vi "Config.vi"(8 "error in":errorcluster, 11 "Instrument Handle In":i32) -> (0 "error out":errorcluster, 2 "Configuration out":i32[](array[numeric]), 3 "Instrument Handle Out":i32)   [LabVIEW 8.6, in "ZTScopeM.lvlib"]
doc: "Query the instrument configuration state."
uses:
  ZTScopeM.lvlib
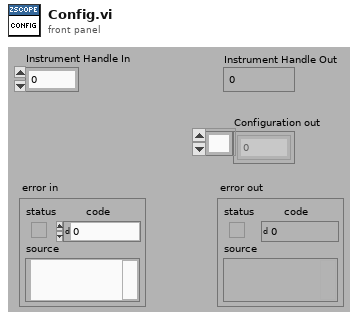
[diagram p1: front panel]
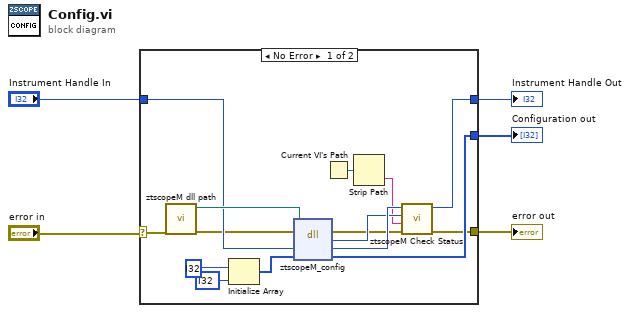
[diagram p0: block diagram]
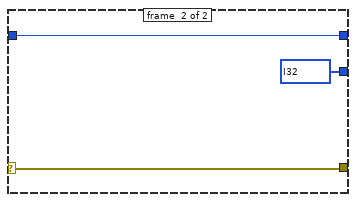
[diagram p2: hidden frame]
diagram:
  n1 = case shown="No Error" "error in" {
    selector: "error in" -> [w10 w23]
    tunnel: [w15 w23] -> w4
    tunnel: [w14 w21] -> w3
    tunnel: [w19 i32[] ? ("Configuration")] -> w2
    tunnel: "Instrument Handle In" -> [w8 w21]
    frame #0 {
      n2 = call "ztscopeM dll path.vi"("error in (no error)"=w10) -> ("error out"=w7:errorcluster, "<instrument>.dll path"=w9:path)  [unwired: 9 in]
      n3 = Initialize Array(i32 ?, i32 ? ("dimension size")) -> (w16:i32[])
      n4 = dll-call lib="C:/Projects/codedepot/Teradyne/2016-1034 Teradyne ZScope API/Software/ZTScopePackageForPVI/PVI VIs/ztscopeM.dll" fn="ztscopeM_config"(path in=w9, error in=w7, "instrumentHandle"=w8, "Configuration"=w16) -> (error out=w6:errorcluster, "return type"=w12:i32, "instrumentHandle"=w13:i32, "Configuration"=w19:i32[])  [unwired: 1 in, 1 out]
      n5 = Current VI's Path() -> (path=w20:path)
      n6 = Strip Path(path=w20) -> (name=w11:string)  [unwired: 1 out]
      n7 = call "ztscopeM Check Status.vi"("error in"=w6, "name of VI"=w11, "status (return code)"=w12, "instrument handle in"=w13) -> ("error out"=w15:errorcluster, "instrument handle out"=w14:i32)  [unwired: 2 in]
    }
    frame #1 {
    }
  }
  "Instrument Handle Out" <- w3
  "error out" <- w4
  "Configuration out" <- w2
